vi "cam0#-搜索铜碎.vi"(8 "Cut基点":cluster{"X":sgl, "Y":sgl}, 9 "输入参数信息":T5, 11 "images":T4) -> (0 "存在铜碎":bool, 1 "检出点":cluster{"X":sgl, "Y":sgl}[](array[cluster]), 3 "ImageOUT":T1, 4 "ImageMorphOut":T1)   [LabVIEW 2015]
uses:
  <vilib>/vision/Image Controls.llb/IMAQ Image.ctl
  <vilib>/vision/NI_Vision_Development_Module.lvlib
panel:
  in  "槽口反光排除带区宽度":sgl=25.0
  out "ImageMorphOut 4":T1
  out "ImageMorphOut 2":T1
  out "错误输出":errorcluster
  out "槽内存在铜碎异常":bool
  out "槽形态断裂情况":i32
  out "槽根部存在铜碎异常":bool
  in  "Keep/Remove Particles (F) 2":bool=TRUE
  in  "Selection Values 2":T3(array[cluster])=[{"Measurement Parameter"=35, "Range Lower Value"=0.0, "Range Upper Value"=50.0, "Range"=FALSE, "Measurement Type"=FALSE}] {"Measurement Parameter" items=["Center of Mass X", "Center of Mass Y", "First Pixel X", "First Pixel Y", "Bounding Rect Left", "Bounding Rect Top", "Bounding Rect Right", "Bounding Rect Bottom", "Max Feret Diameter Start X", "Max Feret Diameter Start Y", "Max Feret Diameter End X", "Max Feret Diameter End Y", "Max Horiz. Segment Length Left", "Max Horiz. Segment Length Right", "Max Horiz. Segment Length Row", "-", "Bounding Rect Width", "Bounding Rect Height", "Bounding Rect Diagonal", "Perimeter", "Convex Hull Perimeter", "Holes' Perimeter", "Max Feret Diameter", "Equivalent Ellipse Major Axis", "Equivalent Ellipse Minor Axis", "Equivalent Ellipse Minor Axis (Feret)", "Equivalent Rect Long Side", "Equivalent Rect Short Side", "Equivalent Rect Diagonal", "Equivalent Rect Short Side (Feret)", "Average Horiz. Segment Length", "Average Vert. Segment Length", "Hydraulic Radius", "Waddel Disk Diameter", "-", "Area", "Holes' Area", "Particle & Holes' Area", "Convex Hull Area", "Image Area", "-", "Number of Holes", "Number of Horiz. Segments", "Number of Vert. Segments", "-", "Orientation", "Max Feret Diameter Orientation", "-", "% Area/Image Area", "% Area/(Particle & Holes' Area)", "Ratio of Equivalent Ellipse Axes", "Ratio of Equivalent Rect Sides", "-", "Elongation Factor", "Compactness Factor", "Heywood Circularity Factor", "Type Factor", "-", "Sum X", "Sum Y", "Sum XX", "Sum XY", "Sum YY", "Sum XXX", "Sum XXY", "Sum XYY", "Sum YYY", "-", "Moment of Inertia XX", "Moment of Inertia XY", "Moment of Inertia YY", "Moment of Inertia XXX", "Moment of Inertia XXY", "Moment of Inertia XYY", "Moment of Inertia YYY", "Norm. Moment of Inertia XX", "Norm. Moment of Inertia XY", "Norm. Moment of Inertia YY", "Norm. Moment of Inertia XXX", "Norm. Moment of Inertia XXY", "Norm. Moment of Inertia XYY", "Norm. Moment of Inertia YYY", "Hu Moment 1", "Hu Moment 2", "Hu Moment 3", "Hu Moment 4", "Hu Moment 5", "Hu Moment 6", "Hu Moment 7"]; "Range Lower Value" format="%.2f"; "Range Upper Value" format="%.2f"}
  out "槽根部断裂型铜碎数量":i32
  in  "Keep/Remove Particles (F)":bool
  in  "Selection Values":T3(array[cluster])=[{"Measurement Parameter"=35, "Range Lower Value"=0.0, "Range Upper Value"=1000.0, "Range"=TRUE, "Measurement Type"=FALSE}] {"Measurement Parameter" items=["Center of Mass X", "Center of Mass Y", "First Pixel X", "First Pixel Y", "Bounding Rect Left", "Bounding Rect Top", "Bounding Rect Right", "Bounding Rect Bottom", "Max Feret Diameter Start X", "Max Feret Diameter Start Y", "Max Feret Diameter End X", "Max Feret Diameter End Y", "Max Horiz. Segment Length Left", "Max Horiz. Segment Length Right", "Max Horiz. Segment Length Row", "-", "Bounding Rect Width", "Bounding Rect Height", "Bounding Rect Diagonal", "Perimeter", "Convex Hull Perimeter", "Holes' Perimeter", "Max Feret Diameter", "Equivalent Ellipse Major Axis", "Equivalent Ellipse Minor Axis", "Equivalent Ellipse Minor Axis (Feret)", "Equivalent Rect Long Side", "Equivalent Rect Short Side", "Equivalent Rect Diagonal", "Equivalent Rect Short Side (Feret)", "Average Horiz. Segment Length", "Average Vert. Segment Length", "Hydraulic Radius", "Waddel Disk Diameter", "-", "Area", "Holes' Area", "Particle & Holes' Area", "Convex Hull Area", "Image Area", "-", "Number of Holes", "Number of Horiz. Segments", "Number of Vert. Segments", "-", "Orientation", "Max Feret Diameter Orientation", "-", "% Area/Image Area", "% Area/(Particle & Holes' Area)", "Ratio of Equivalent Ellipse Axes", "Ratio of Equivalent Rect Sides", "-", "Elongation Factor", "Compactness Factor", "Heywood Circularity Factor", "Type Factor", "-", "Sum X", "Sum Y", "Sum XX", "Sum XY", "Sum YY", "Sum XXX", "Sum XXY", "Sum XYY", "Sum YYY", "-", "Moment of Inertia XX", "Moment of Inertia XY", "Moment of Inertia YY", "Moment of Inertia XXX", "Moment of Inertia XXY", "Moment of Inertia XYY", "Moment of Inertia YYY", "Norm. Moment of Inertia XX", "Norm. Moment of Inertia XY", "Norm. Moment of Inertia YY", "Norm. Moment of Inertia XXX", "Norm. Moment of Inertia XXY", "Norm. Moment of Inertia XYY", "Norm. Moment of Inertia YYY", "Hu Moment 1", "Hu Moment 2", "Hu Moment 3", "Hu Moment 4", "Hu Moment 5", "Hu Moment 6", "Hu Moment 7"]}
  # "180110a-初始版本-测量槽宽"
  # "180126a-将基于边沿检测的铜碎搜索方法改为基于形态学的处理方法"
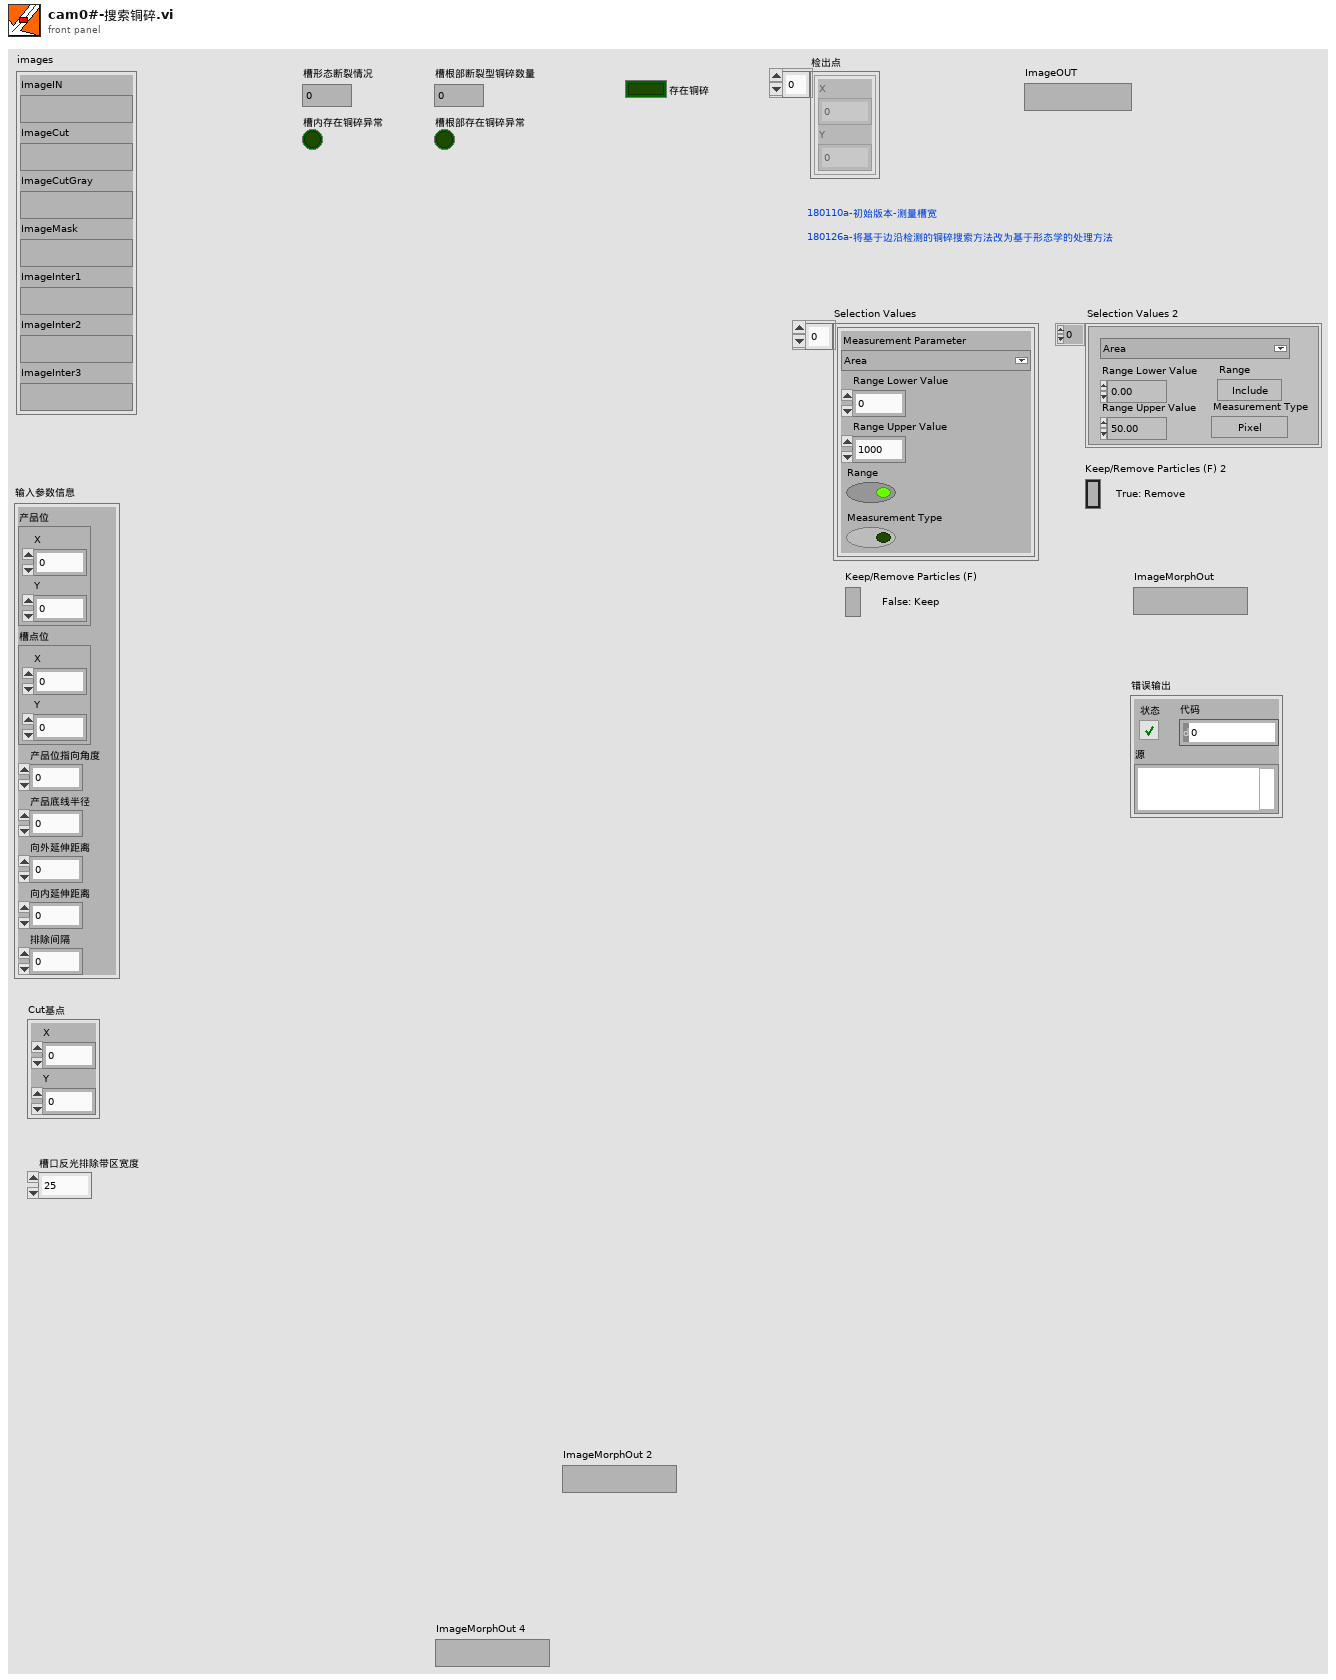
[diagram p1: front panel]
types:
  T1 = typedef "IMAQ Image.ctl" = refnum<image>
  T2 = typedef "Particle Parameters" = i32
  T3 = cluster{"Measurement Parameter":T2, "Range Lower Value":dbl, "Range Upper Value":dbl, "Range":bool, "Measurement Type":bool}[]
  T4 = cluster{"ImageIN":T1, "ImageCut":T1, "ImageCutGray":T1, "ImageMask":T1, "ImageInter1":T1, "ImageInter2":T1, "ImageInter3":T1}
  T5 = cluster{"产品位":cluster{"X":sgl, "Y":sgl}, "槽点位":cluster{"X":sgl, "Y":sgl}, "产品位指向角度":sgl, "产品底线半径":sgl, "向外延伸距离":sgl, "向内延伸距离":sgl, "排除间隔":sgl}
  T6 = typedef "IMAQ Circle" = cluster{"Center X":i32, "Center Y":i32, "Inner Radius":i32, "Outer Radius":i32, "Start Angle":dbl, "End Angle":dbl}
  T7 = enum32{"Average", "Min", "Max", "Clear  if < ", "Clear  if < or =", "Clear  if =", "Clear  if > or =", "Clear  if >"}
  T8 = enum32{"AutoM", "Close", "Dilate", "Erode", "Gradient", "Gradient out", "Gradient in", "Hit miss", "Open", "PClose", "POpen", "Thick", "Thin"}
  T9 = typedef "ROI Descriptor" = cluster{"Global Rectangle":i32[], "Contours":cluster{"ID":enum32{"External", "Internal"}, "Type":u32, "Coordinates":i32[]}[]}
  T10 = cluster{"Mean Intensity":sgl, "Standard  Deviation":sgl, "Minimum Intensity":sgl, "Maximum Intensity":sgl}
  T11 = cluster{"Starting Value":sgl, "Interval Width":sgl, "histogram":u32[]}
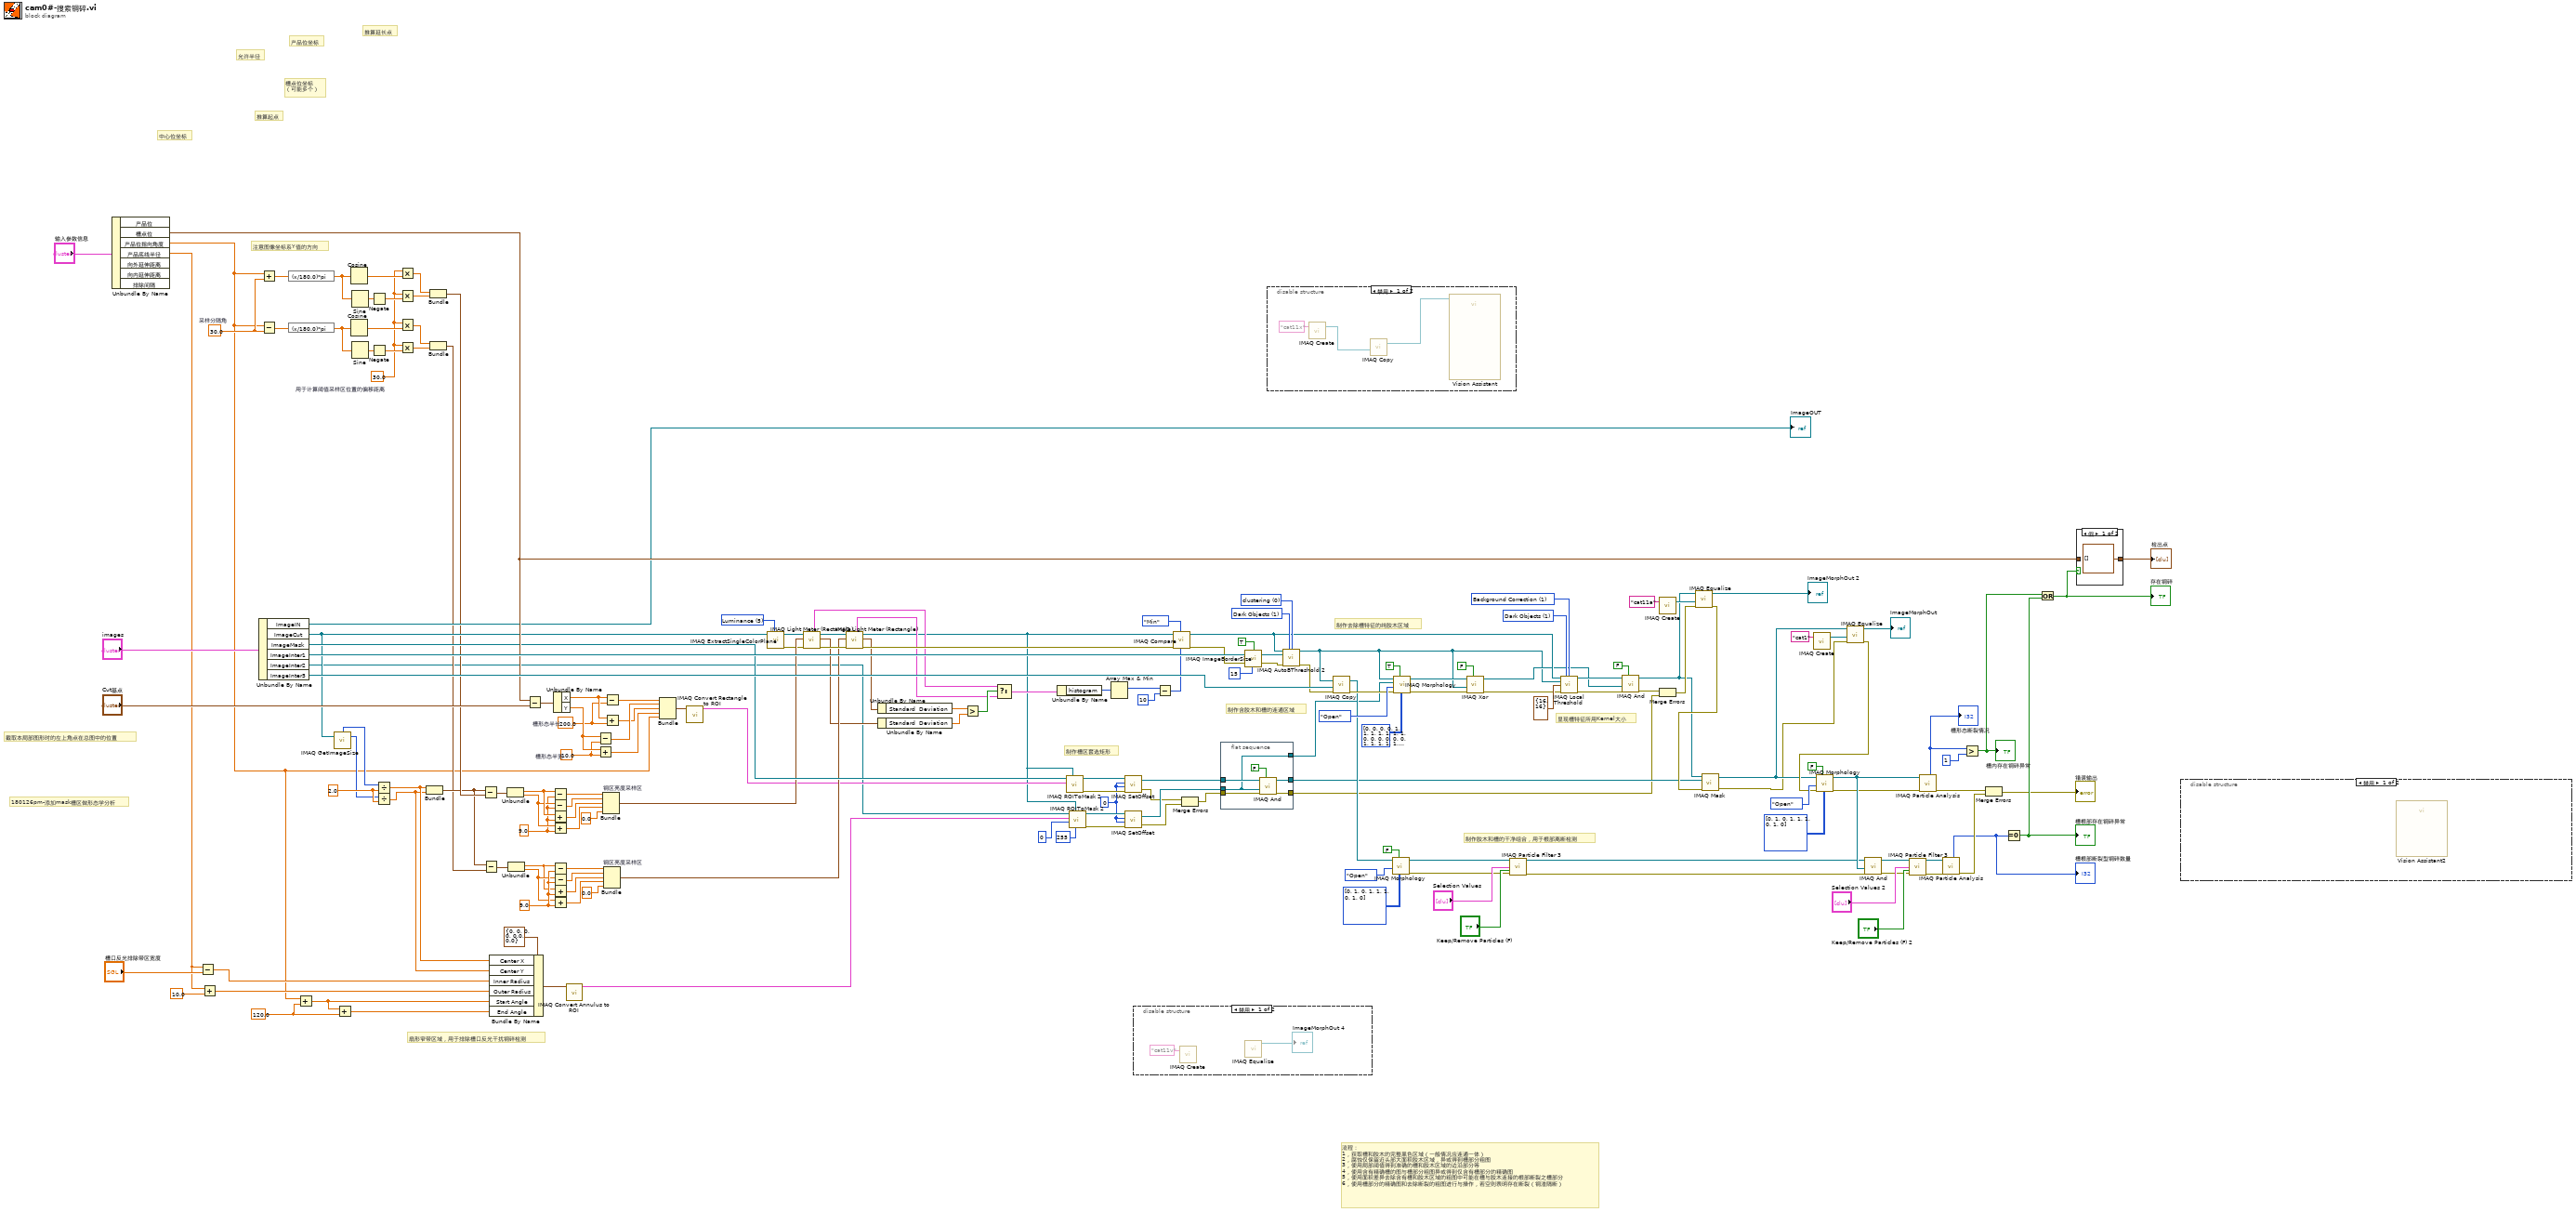
[diagram p0: block diagram]
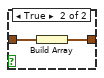
[diagram p4: hidden frame]
diagram:
  w15 = 0 ("X Offset")
  w37 = 120.0 ("y")
  w75 = sgl 9.0 ("y")
  w81 = sgl 30.0  # 采样分隔角
  w109 = 2.0 ("y")
  w115 = sgl 9.0 ("y")
  w83 = sgl 30.0  # 用于计算阈值采样区位置的偏移距离
  w155 = u32 1 items=["Bright Objects", "Dark Objects"] ("Look For (Bright Objects)")
  w157 = u32 1 items=["Niblack", "Background Correction"] ("Method")
  w161 = 0 items=["clustering", "entropy", "metric", "moments", "inter-class variance"] ("Method")
  w162 = u32 1 items=["Bright Objects", "Dark Objects"] ("Look For")
  w164 = 5 items=["Red", "Green", "Blue", "Hue", "Saturation", "Luminance", "Value", "Intensity"] ("Color Plane")
  w166 = sgl 200.0  # 槽形态半长
  w176 = sgl 10.0  # 槽形态半宽
  # "扇形窄带区域，用于排除槽口反光干扰铜碎检测"
  # "截取本局部图形时的左上角点在总图中的位置"
  # "显现槽特征所用Kernel大小"
  # "制作去除槽特征的纯胶木区域"
  # "制作含胶木和槽的连通区域"
  # "制作胶木和槽的干净组合，用于根部离断检测"
  # "制作槽区套选矩形"
  # "流程：\n1，获取槽和胶木的完整黑色区域（一般情况应连通一体）\n2，腐蚀仅保留近头部大面积胶木区域，异或得到槽部分粗图\n3，使用局部阈值得到准确的槽和胶木区域的边沿部分等\n4，使用含有精确槽的图与槽部分粗图异或得到仅含有槽部分的精确图\n5，使用面积差异去除含有槽和胶木区域的粗图中可能在槽与胶木连接的根部断裂之槽部分\n6，使用槽部分的精确图和去除断裂的粗图进行与操作，若空则表明存在断裂（铜渣隔断）"
  # "180126pm-添加mask槽区做形态学分析"
  # "注意图像坐标系Y值的方向"
  # "允许半径"
  # "推算起点"
  # "推算延长点"
  # "槽点位坐标\n（可能多个）"
  # "产品位坐标"
  # "中心位坐标"
  n1 = Unbundle By Name("输入参数信息") -> ("槽点位"=w126:cluster{"X":sgl, "Y":sgl}, "产品位指向角度"=w36:sgl, "产品底线半径"=w40:sgl)  [unwired: 4 out]
  n2 = Subtract(x=w40, y="槽口反光排除带区宽度") -> (x-y=w41:sgl)
  n3 = Add(x=w40, y=sgl 10.0) -> (x+y=w38:sgl)
  n4 = Unbundle By Name("images") -> ("ImageIN"=→"ImageOUT":T1, "ImageCut"=w106:T1, "ImageMask"=w123:T1, "ImageInter1"=w150:T1, "ImageInter2"=w4:T1, "ImageInter3"=w147:T1)
  n5 = Add(x=w36, y=w81) -> (x+y=w90:sgl)
  n6 = Subtract(x=w36, y=w81) -> (x-y=w82:sgl)
  n7 = expression code="(x/180.0)*pi" ("degrees to radians")(w90) -> (w181:sgl)
  n8 = expression code="(x/180.0)*pi" ("degrees to radians")(w82) -> (w84:sgl)
  n9 = Add(x=w36, y=w37) -> (x+y=w33:dbl)
  n10 = call "IMAQ GetImageSize"("Image"=w106) -> ("Y Resolution"=w107:i32, "X Resolution"=w108:i32)  [unwired: 3 in, 1 out]
  n11 = Add(x=w33, y=w37) -> (x+y=w35:dbl)
  n12 = Cosine(x=w181) -> (cos(x)=w120:sgl)
  n13 = Cosine(x=w84) -> (cos(x)=w88:sgl)
  n14 = Sine(x=w181) -> (sin(x)=w179:sgl)
  n15 = Sine(x=w84) -> (sin(x)=w85:sgl)
  n16 = Negate(x=w179) -> (-x=w119:sgl)
  n17 = Negate(x=w85) -> (-x=w89:sgl)
  n18 = Divide(x=w108, y=w109) -> (x/y=w44:dbl)
  n19 = Divide(x=w107, y=w109) -> (x/y=w43:dbl)
  n20 = Multiply(x=w83, y=w120) -> (x*y=w122:sgl)
  n21 = Multiply(x=w83, y=w119) -> (x*y=w121:sgl)
  n22 = Multiply(x=w83, y=w88) -> (x*y=w86:sgl)
  n23 = Multiply(x=w83, y=w89) -> (x*y=w87:sgl)
  n24 = Bundle(w44, w43) -> (w70:cluster{dbl, dbl})  [unwired: 1 in]
  n25 = Bundle(w122, w121) -> (w71:cluster{sgl, sgl})  [unwired: 1 in]
  n26 = Bundle(w86, w87) -> (w69:cluster{sgl, sgl})  [unwired: 1 in]
  n27 = Subtract(x=w70, y=w71) -> (x-y=w118:cluster{dbl, dbl})
  n28 = Subtract(x=w70, y=w69) -> (x-y=w72:cluster{dbl, dbl})
  n29 = Bundle By Name(cluster=T6 {"Center X"=0, "Center Y"=0, "Inner Radius"=0, "Outer Radius"=0, "Start Angle"=0.0, "End Angle"=0.0} ("Annulus"), "Center X"=w44, "Center Y"=w43, "Inner Radius"=w41, "Outer Radius"=w38, "Start Angle"=w33, "End Angle"=w35) -> (w45:T6)
  n30 = Unbundle(w118) -> (w117:dbl, w116:dbl)
  n31 = Unbundle(w72) -> (w73:dbl, w74:dbl)
  n32 = Subtract(x=w126, y="Cut基点") -> (x-y=w167:cluster{"X":sgl, "Y":sgl})
  n33 = Subtract(x=w117, y=w115) -> (x-y=w114:dbl)
  n34 = Subtract(x=w116, y=w115) -> (x-y=w113:dbl)
  n35 = Add(x=w117, y=w115) -> (x+y=w112:dbl)
  n36 = Add(x=w116, y=w115) -> (x+y=w111:dbl)
  n37 = Subtract(x=w73, y=w75) -> (x-y=w76:dbl)
  n38 = Subtract(x=w74, y=w75) -> (x-y=w77:dbl)
  n39 = Add(x=w73, y=w75) -> (x+y=w78:dbl)
  n40 = Add(x=w74, y=w75) -> (x+y=w79:dbl)
  n41 = Unbundle By Name(w167) -> ("X"=w178:sgl, "Y"=w177:sgl)
  n42 = call "IMAQ Convert Annulus to ROI"("Annulus"=w45) -> ("ROI Descriptor"=w31:T9)  [unwired: 8 in, 1 out]
  n43 = Subtract(x=w177, y=w176) -> (x-y=w174:sgl)
  n44 = Add(x=w177, y=w176) -> (x+y=w172:sgl)
  n45 = Bundle "铜区亮度采样区"(w114, w113, w112, w111, "y"=sgl 0.0) -> (w104:cluster{dbl, dbl, dbl, dbl, "y":sgl})  [unwired: 1 in]
  n46 = Bundle "铜区亮度采样区"(w76, w77, w78, w79, "y"=sgl 0.0) -> (w65:cluster{dbl, dbl, dbl, dbl, "y":sgl})  [unwired: 1 in]
  n47 = Subtract(x=w178, y=w166) -> (x-y=w175:sgl)
  n48 = Add(x=w178, y=w166) -> (x+y=w173:sgl)
  n49 = Bundle(w175, w174, w173, w172, "产品位指向角度"=w36) -> (w170:cluster{sgl, sgl, sgl, sgl, "产品位指向角度":sgl})  [unwired: 1 in]
  n50 = call "IMAQ Convert Rectangle to ROI"("Rectangle"=w170) -> ("ROI Descriptor"=w34:T9)  [unwired: 8 in, 1 out]
  n51 = call "IMAQ ExtractSingleColorPlane"("Color Plane"=w164, "Image Src"=w106) -> ("error out"=w92:errorcluster, "Image Dst Out"=w98:T1)  [unwired: 8 in]
  n52 = call "IMAQ Light Meter (Rectangle)"("error in (no error)"=w92, "Rectangle"=w104, "Image"=w98) -> ("error out"=w67:errorcluster, "Gray Level Intensities"=w63:T10, "Image Out"=w68:T1, "Histogram"=w59:T11)  [unwired: 4 in, 1 out]
  n53 = call "IMAQ Light Meter (Rectangle)"("error in (no error)"=w67, "Rectangle"=w65, "Image"=w68) -> ("error out"=w66:errorcluster, "Gray Level Intensities"=w64:T10, "Image Out"=w2:T1, "Histogram"=w58:T11)  [unwired: 4 in, 1 out]
  n54 = Unbundle By Name(w64) -> ("Standard  Deviation"=w62:sgl)
  n55 = Unbundle By Name(w63) -> ("Standard  Deviation"=w61:sgl)
  n56 = Greater?(x=w62, y=w61) -> (0:w60:bool)
  n57 = Select(t=w59, s=w60, f=w58) -> (s? t:f=w57:T11)
  n58 = Unbundle By Name(w57) -> ("histogram"=w102:u32[])
  n59 = call "IMAQ ROIToMask 2"("Image Model"=w2, "ROI Descriptor"=w34, "Image"=w123) -> ("error out"=w168:errorcluster, "Image Out"=w169:T1)  [unwired: 6 in, 1 out]
  n60 = call "IMAQ ROIToMask 2"("Background Value (0)"=255, "Image Model"=w2, "Filling Value (255)"=0, "ROI Descriptor"=w31, "Image"=w4) -> ("error out"=w32:errorcluster, "Image Out"=w30:T1)  [unwired: 4 in, 1 out]
  n61 = Array Max & Min(array=w102) -> (max index (indices)=w99:i32)  [unwired: 3 out]
  n62 = call "IMAQ SetOffset"("error in (no error)"=w168, "Y Offset"=w15, "X Offset"=w15, "Image"=w169) -> ("error out"=w8:errorcluster, "Image Out"=w10:T1)
  n63 = call "IMAQ SetOffset"("error in (no error)"=w32, "Y Offset"=w15, "X Offset"=w15, "Image"=w30) -> ("error out"=w7:errorcluster, "Image Out"=w13:T1)
  n64 = disable-structure shown="禁用" {
    frame Disabled {
      n65 = call "IMAQ Create"("Image Name"="cat11v") -> ()  [unwired: 4 in, 2 out]
      n66 = call "IMAQ Equalize"() -> ("Image Dst Out"=→"ImageMorphOut 4":T1)  [unwired: 10 in, 1 out]
    }
    frame Enabled {
    }
  }
  n67 = Subtract(x=w99, y=u32 10) -> (x-y=w100:u32)
  n68 = call "IMAQ Compare"("Constant"=w100, "Operator"=T7."Min", "error in (no error)"=w66, "Image Src A"=w2) -> ("error out"=w103:errorcluster, "Image Dst Out"=w47:T1)  [unwired: 6 in]
  n69 = Merge Errors(w8, w7) -> (w6:errorcluster)
  n70 = flat-sequence {
    tunnel: w13 -> [w184]
    tunnel: w10 -> [w188]
    tunnel: [w187] -> w9
    tunnel: w6 -> [w186]
    tunnel: [w185] -> w5
    tunnel: [w184] -> w3
    frame #0 {
      n71 = call "IMAQ And"("And/Nand (And)"=FALSE, "error in (no error)"=w186, "Image Src B"=w184, "Image Src A"=w188) -> ("error out"=w185:errorcluster, "Image Dst Out"=w187:T1)  [unwired: 2 in, 4 out]
    }
  }
  n72 = call "IMAQ ImageBorderSize"("Get/Set Status? (Set)"=TRUE, "Image"=w150, "Image border size in"=15 ("Border Size"), "error in (no error)"=w103) -> ("Image Out"=w149:T1, "error out"=w151:errorcluster)  [unwired: 1 out]
  n73 = disable-structure shown="禁用" {
    frame Disabled {
      n74 = call "IMAQ Create"("Image Name"="cat11x") -> ("New Image"=w191:T1)  [unwired: 4 in, 1 out]
      n75 = call "IMAQ Copy"("Image Dst"=w191) -> ("Image Dst Out"=w190:T1)  [unwired: 5 in, 1 out]
      n76 = call "Vision Assistant"("Image In"=w190) -> ()  [unwired: 25 in, 2 out]
    }
    frame Enabled {
    }
  }
  n77 = call "IMAQ AutoBThreshold 2"("Image Src"=w47, "Look For (Bright Objects)"=w162, "Method (clustering)"=w161, "Image Dst"=w149, "error in (no error)"=w151) -> ("Image Dst Out"=w24:T1, "error out"=w1:errorcluster)  [unwired: 3 in, 6 out]
  n78 = call "IMAQ Copy"("error in (no error)"=w1, "Image Dst"=w147, "Image Src"=w24) -> ("error out"=w148:errorcluster, "Image Dst Out"=w49:T1)  [unwired: 3 in]
  n79 = call "IMAQ Morphology"("Structuring Element"=i32[][] [[0, 1, 0], [1, 1, 1], [0, 1, 0]], "Square/Hexa (Square)"=FALSE, "Operation"=T8."Open", "Image Src"=w49) -> ("error out"=w141:errorcluster, "Image Dst Out"=w50:T1)  [unwired: 6 in]
  n80 = call "IMAQ Morphology"("Structuring Element"=i32[][] [[0, 0, 0, 0, 1, 1, 1, 1, 1, 1, 1, 0, 0, 0, 0], [0, 0, 1, 1, 1, 1, 1, 1, 1, 1, 1, 1, 1, 0, 0], [0, 1, 1, 1, 1, 1, 1, 1, 1, 1, 1, 1, 1, 1, 0], [0, 1, 1, 1, 1, 1, 1, 1, 1, 1, 1, 1, 1, 1, 0], [1, 1, 1, 1, 1, 1, 1, 1, 1, 1, 1, 1, 1, 1, 1], [1, 1, 1, 1, 1, 1, 1, 1, 1, 1, 1, 1, 1, 1, 1], [1, 1, 1, 1, 1, 1, 1, 1, 1, 1, 1, 1, 1, 1, 1], [1, 1, 1, 1, 1, 1, 1, 1, 1, 1, 1, 1, 1, 1, 1], [1, 1, 1, 1, 1, 1, 1, 1, 1, 1, 1, 1, 1, 1, 1], [1, 1, 1, 1, 1, 1, 1, 1, 1, 1, 1, 1, 1, 1, 1], [1, 1, 1, 1, 1, 1, 1, 1, 1, 1, 1, 1, 1, 1, 1], [0, 1, 1, 1, 1, 1, 1, 1, 1, 1, 1, 1, 1, 1, 0], [0, 1, 1, 1, 1, 1, 1, 1, 1, 1, 1, 1, 1, 1, 0], [0, 0, 1, 1, 1, 1, 1, 1, 1, 1, 1, 1, 1, 0, 0], [0, 0, 0, 0, 1, 1, 1, 1, 1, 1, 1, 0, 0, 0, 0]] ("Structuring Element (Basic Morphology 2)"), "Square/Hexa (Square)"=TRUE, "error in (no error)"=w148, "Operation"=T8."Open", "Image Dst"=w3, "Image Src"=w24) -> ("error out"=w14:errorcluster, "Image Dst Out"=w25:T1)  [unwired: 1 in, 3 out]
  n81 = call "IMAQ Xor"("Xor/Xnor (Xor)"=FALSE, "error in (no error)"=w14, "Image Src B"=w24, "Image Src A"=w25) -> ("error out"=w26:errorcluster, "Image Dst Out"=w27:T1)  [unwired: 2 in, 4 out]
  n82 = call "IMAQ Particle Filter 3"("Image Src"=w50, "Selection Values"="Selection Values", "Keep/Remove Particles (F)"="Keep/Remove Particles (F)", "error in (no error)"=w141) -> ("Image Dst Out"=w51:T1, "error out"=w55:errorcluster)  [unwired: 9 in, 1 out]
  n83 = call "IMAQ Local Threshold"("Image Src"=w47, "Look For (Bright Objects)"=w155, "Method (Niblack)"=w157, "Image Dst"=w24, "Window Size (32x32)"=cluster{"SizeX":i32, "SizeY":i32} {"SizeX"=16, "SizeY"=16} ("Kernel Size"), "error in (no error)"=w26) -> ("Image Dst Out"=w28:T1, "error out"=w22:errorcluster)  [unwired: 2 in, 6 out]
  n84 = call "IMAQ And"("And/Nand (And)"=FALSE, "error in (no error)"=w22, "Image Src B"=w27, "Image Src A"=w28) -> ("error out"=w56:errorcluster, "Image Dst Out"=w19:T1)  [unwired: 2 in, 4 out]
  n85 = call "IMAQ Create"("Image Name"="cat11a") -> ("New Image"=w54:T1)  [unwired: 4 in, 1 out]
  n86 = Merge Errors(w56, w5) -> (w21:errorcluster)
  n87 = call "IMAQ Equalize"("error in (no error)"=w21, "Image Dst"=w54, "Image Src"=w19) -> ("error out"=w20:errorcluster, "Image Dst Out"=→"ImageMorphOut 2":T1)  [unwired: 7 in]
  n88 = call "IMAQ Mask"("error in (no error)"=w20, "Image Mask"=w9, "Image Src"=w19) -> ("error out"=w11:errorcluster, "Image Dst Out"=w12:T1)  [unwired: 2 in]
  n89 = call "IMAQ Create"("Image Name"="cat1") -> ("New Image"=w95:T1)  [unwired: 4 in, 1 out]
  n90 = call "IMAQ Equalize"("error in (no error)"=w11, "Image Dst"=w95, "Image Src"=w12) -> ("error out"=w17:errorcluster, "Image Dst Out"=→"ImageMorphOut":T1)  [unwired: 7 in]
  n91 = call "IMAQ Morphology"("Structuring Element"=i32[][] [[0, 1, 0], [1, 1, 1], [0, 1, 0]], "Square/Hexa (Square)"=FALSE, "error in (no error)"=w17, "Operation"=T8."Open", "Image Src"=w12) -> ("error out"=w18:errorcluster, "Image Dst Out"=w94:T1)  [unwired: 5 in]
  n92 = call "IMAQ And"("error in (no error)"=w55, "Image Src B"=w94, "Image Src A"=w51) -> ("error out"=w135:errorcluster, "Image Dst Out"=w48:T1)  [unwired: 3 in, 4 out]
  n93 = call "IMAQ Particle Filter 3"("Image Src"=w48, "Selection Values"="Selection Values 2", "Keep/Remove Particles (F)"="Keep/Remove Particles (F) 2", "error in (no error)"=w135) -> ("Image Dst Out"=w136:T1, "error out"=w139:errorcluster)  [unwired: 9 in, 1 out]
  n94 = call "IMAQ Particle Analysis"("error in (no error)"=w18, "Image"=w94) -> ("error out"=w131:errorcluster, "Number of Particles"=w130:i32)  [unwired: 4 in, 4 out]
  "槽形态断裂情况" <- w130
  n95 = call "IMAQ Particle Analysis"("error in (no error)"=w139, "Image"=w136) -> ("error out"=w140:errorcluster, "Number of Particles"=w97:i32)  [unwired: 4 in, 4 out]
  "槽根部断裂型铜碎数量" <- w97
  n96 = Greater?(x=w130, y=1) -> (0:w128:bool)
  "槽内存在铜碎异常" <- w128
  n97 = Merge Errors(w131, w140) -> (→"错误输出":errorcluster)
  n98 = Equal To 0?(x=w97) -> (x = 0?=w127:bool)
  "槽根部存在铜碎异常" <- w127
  n99 = Or(x=w128, y=w127) -> (x .or. y?=w124:bool)
  "存在铜碎" <- w124
  n100 = case shown="假" w124 {
    tunnel: w126 -> [_ w195]
    tunnel: [cluster{"X":sgl, "Y":sgl}[] [] w194] -> w125
    frame False {
    }
    frame True {
      n101 = Build Array(w195) -> (w194:cluster{"X":sgl, "Y":sgl}[])
    }
  }
  "检出点" <- w125
  n102 = disable-structure shown="禁用" {
    frame Disabled {
      n103 = call "Vision Assistant2"() -> ()  [unwired: 25 in, 3 out]
    }
    frame Enabled {
    }
  }
